vi "test-linear-filter-test-03-derivE.vi"(11 "Input":dbl) -> (3 "Output":dbl)   [LabVIEW 2019]
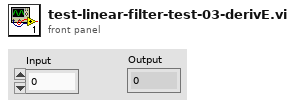
[diagram p1: front panel]
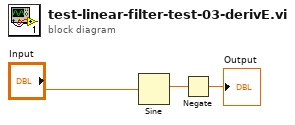
[diagram p0: block diagram]
diagram:
  n1 = Sine(x="Input") -> (sin(x)=w2:dbl)
  n2 = Negate(x=w2) -> (-x=→"Output":dbl)
